vi "MAC_Query.vi"(0 "System no.":i32=1 min=1 max=4 step=1, 2 "Macro name":string, 3 "Get contents?":bool, 5 "error in":errorcluster) -> (14 "Macro names or contents":string, 19 "error out":errorcluster)   [LabVIEW 2020]
doc: "If Get contents? is FALSE, returns names of all available macros, if TRUE, returns contents of one specified macro. \n\nE-816: This command cannot be issued to a slave. Check controller manual to find out if MAC? is supported.\n\nM-8X0: Only for GCS syntax version = GCS 2.0 or higher (check with CSV?.vi. If CSV?.vi is not supported, syntax version is GCS 1.0)."
panel:
  # "If \"Get contents?\" is FALSE, returns names of all available\nmacros, if TRUE, returns contents of one specified macro."
  # "If Get contents = TRUE:"
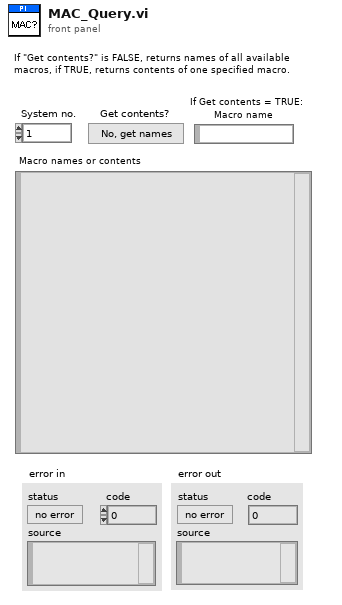
[diagram p1: front panel]
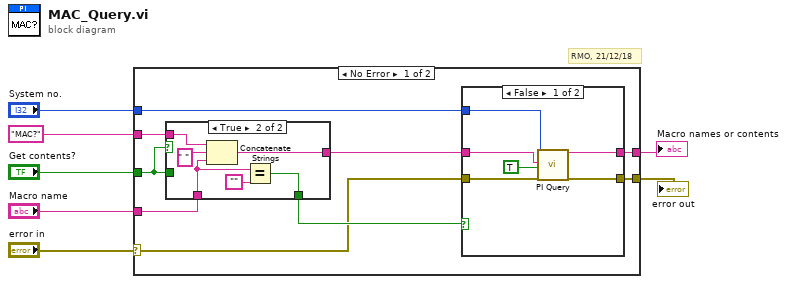
[diagram p0: block diagram]
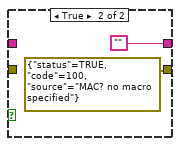
[diagram p2: hidden frame]
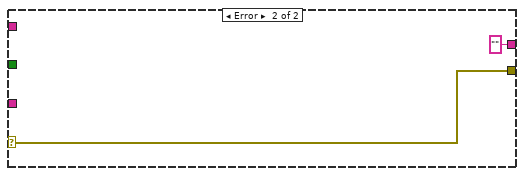
[diagram p4: hidden frame]
diagram:
  # "RMO, 21/12/18"
  n1 = case shown="No Error" "error in" {
    selector: "error in" -> [w8 w33]
    tunnel: [w16 "" ("String read")] -> w7
    tunnel: [w15 w33] -> w6
    tunnel: "System no." -> [w14 _]
    tunnel: "MAC?" ("String to Send") -> [w13 _]
    tunnel: "Macro name" -> [w12 _]
    tunnel: "Get contents?" -> [w11 _]
    frame No Error {
      n2 = case shown="True" w11 {
        tunnel: w13 -> [w26 w32]
        tunnel: w12 -> [_ w28]
        tunnel: [w26 w30] -> w10
        tunnel: [w25 w27] -> w9
        tunnel: w11 -> [w25 _]
        frame False {
        }
        frame True {
          n3 = Concatenate Strings(w32, " ", w28) -> (w30:string)
          n4 = Equal?(x=w28, y="") -> (x = y?=w27:bool)
        }
      }
      n5 = case shown="False" w9 {
        tunnel: [w17 ""] -> w16
        tunnel: [w18 errorcluster {"status"=TRUE, "code"=100, "source"="MAC? no macro specified"} ("error out")] -> w15
        tunnel: w14 -> [w20 _]
        tunnel: w8 -> [w21 _]
        tunnel: w10 -> [w19 _]
        frame False {
          n6 = call "PI Query.vi"("System no."=w20, "String to send"=w19, "Attach termination char.?"=TRUE ("Attach Linefeed?"), "error in"=w21) -> ("String read"=w17:string, "error out"=w18:errorcluster)  [unwired: 3 in, 11 out]
        }
        frame True {
        }
      }
    }
    frame Error {
    }
  }
  "Macro names or contents" <- w7
  "error out" <- w6
